vi "Read Series CFG.vi"(8 "error in":errorcluster, 10 "Series CFG File Path":path, 11 "File Provider in":refnum<class "File Provider.lvclass">) -> (0 "error out":errorcluster, 3 "File Provider out":refnum<class "File Provider.lvclass">)   [LabVIEW 2023, in "File Provider.lvlib" / "File Provider.lvclass"]
uses:
  File Provider.lvclass
  File Provider.lvclass/File Provider.ctl
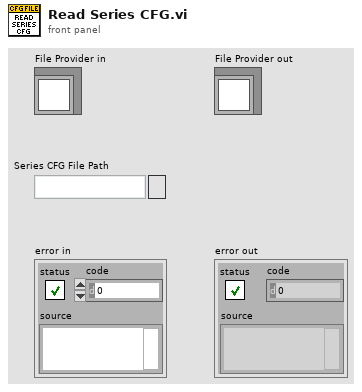
[diagram p1: front panel]
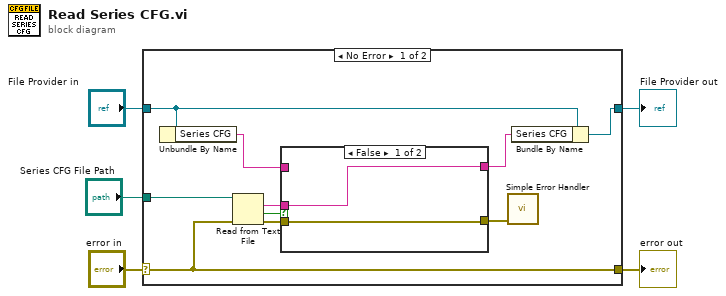
[diagram p0: block diagram]
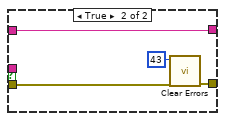
[diagram p2: hidden frame]
diagram:
  n1 = case shown="No Error" "error in" {
    selector: "error in" -> [w6 w23]
    tunnel: [w6 w23] -> w4
    tunnel: [w10 w22] -> w2
    tunnel: "File Provider in" -> [w8 w22]
    tunnel: "Series CFG File Path" -> [w15 _]
    frame No Error {
      n2 = Unbundle By Name(w8) -> ("Series CFG"=w7:string)
      n3 = Read from Text File(file (use dialog)=w15, error in=w6) -> (text=w11:string, cancelled=w14:bool, error out=w13:errorcluster)  [unwired: 2 in, 1 out]
      n4 = case shown="False" w14 {
        tunnel: w13 -> [w16 w21]
        tunnel: [w16 w19] -> w12
        tunnel: w11 -> [w17 _]
        tunnel: [w17 w18] -> w9
        tunnel: w7 -> [_ w18]
        frame False {
        }
        frame True {
          n5 = call <vilib>:"Clear Errors.vi"("error in (no error)"=w21, "specific error code to clear (0: all)"=43) -> ("error out"=w19:errorcluster)  [unwired: 4 in, 1 out]
        }
      }
      n6 = call <vilib>:"Simple Error Handler.vi"("error in (no error)"=w12) -> ()  [unwired: 4 in, 5 out]
      n7 = Bundle By Name(cluster=w8, "Series CFG"=w9) -> (w10:refnum<class "File Provider.lvclass">)
    }
    frame Error {
    }
  }
  "error out" <- w4
  "File Provider out" <- w2
